vi "Cholesky decomposition LABVIEW_v1.3.vi"() -> ()   [LabVIEW 2020]
uses:
  <vilib>/Analysis/Matrix/Datatypes/RealMatrix.ctl
  <vilib>/Analysis/baseanly.llb/Real A x B.vi
  <vilib>/Analysis/7linalg.llb/Real Cholesky Factorization.vi
  <vilib>/Analysis/7linalg.llb/Real Transpose Matrix.vi
  <vilib>/Analysis/baseanly.llb/Full Cholesky Factorization.vi
  <vilib>/Analysis/baseanly.llb/Full Real Matrix Cholesky Factorization.vi
  <vilib>/Analysis/Matrix/Numeric/Subtract/Subtract - RM,RM.vi
  <vilib>/Analysis/NI_AALPro.lvlib
  <vilib>/Analysis/Matrix/NI_Matrix.lvlib
  <vilib>/Analysis/NI_AALBase.lvlib
panel:
  out "sum of error":dbl
  out "error":i32
  out "L LABVIEW-FPGA":sgl[][](array[numeric])
  out "L LABVIEW":T1
  out "A input":dbl[][](array[numeric])
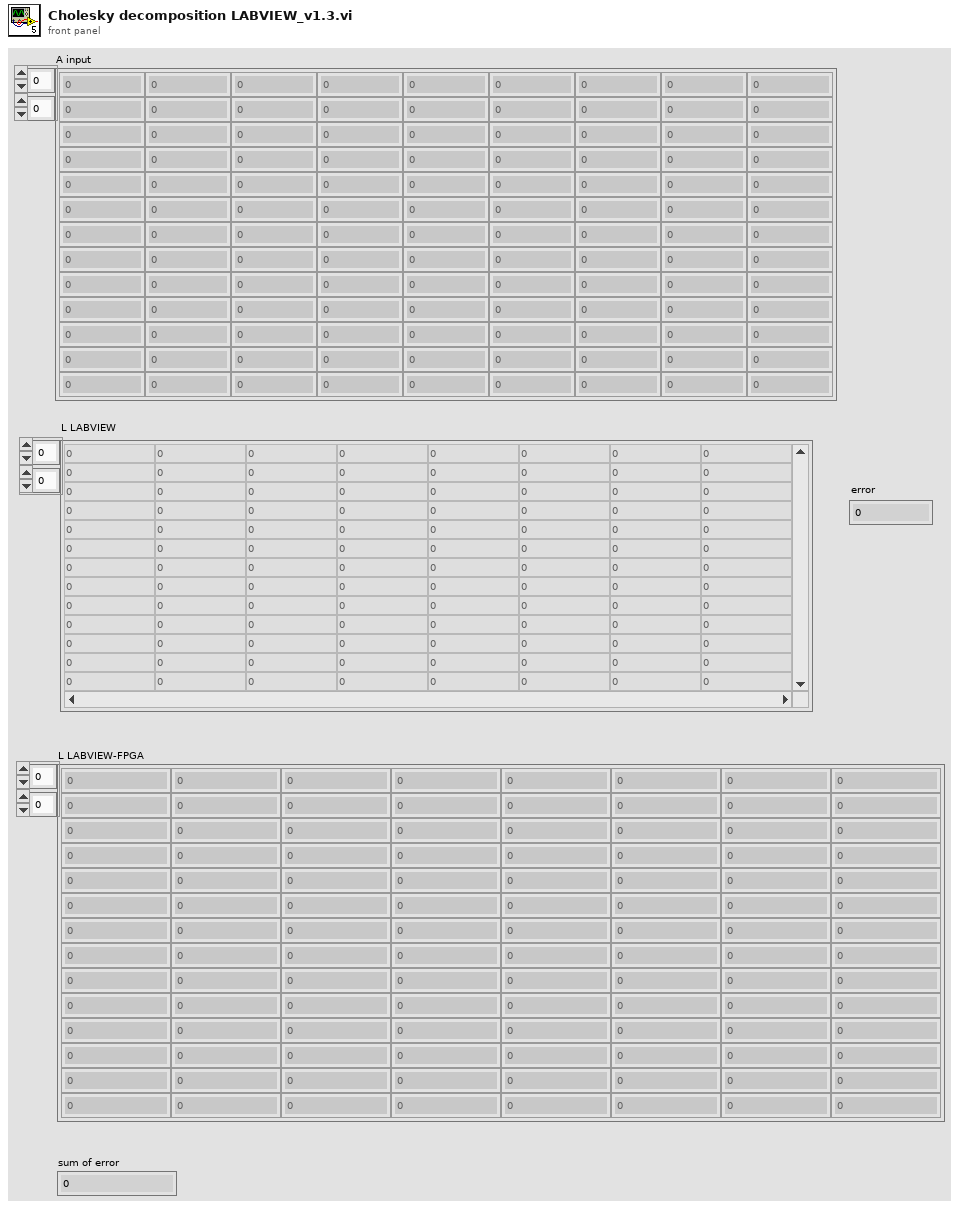
[diagram p1: front panel]
types:
  T1 = typedef "NI_Matrix.lvlib/RealMatrix.ctl" = dbl[][]
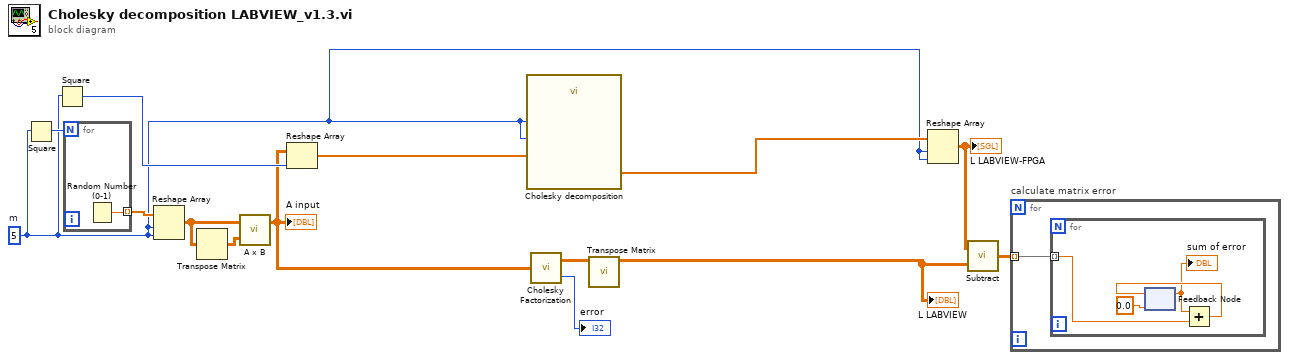
[diagram p0: block diagram]
diagram:
  w1 = 5  # m
  n1 = Square(x=w1) -> (x^2=w6:i32)
  n2 = Square(x=w1) -> (x^2=w11:i32)
  n3 = for {
    N: w6 -> [_]
    tunnel: [w15] -> w5 mode=indexing
    n4 = Random Number (0-1)() -> (number: 0 to 1=w15:dbl)
  }
  n5 = Reshape Array(w5, w1, w1) -> (w3:dbl[][])
  n6 = Transpose Matrix(1:w3) -> (0:w4:dbl[][])
  n7 = call-poly <vilib>:"A x B.vi"("B"=w4, "A"=w3) -> ("A x B"=w2:T1)  [unwired: 1 out]
  "A input" <- w2
  n8 = Reshape Array(w2, w11) -> (w14:dbl[])
  n9 = call "Cholesky decomposition.vi"("n"=w1, "m"=w1, "A"=w14) -> ("L"=w13:sgl[])
  n10 = call-poly <vilib>:"Cholesky Factorization.vi"("A"=w2) -> ("Cholesky"=w10:T1, "error"=→"error":i32)
  n11 = call-poly <vilib>:"Transpose Matrix.vi"("Input Matrix"=w10) -> ("Matrix Transpose"=w7:T1)  [unwired: 9 in, 1 out]
  "L LABVIEW" <- w7
  n12 = Reshape Array(w13, w1, w1) -> (w8:sgl[][])
  "L LABVIEW-FPGA" <- w8
  n13 = call-poly <vilib>:"Subtract.vi"("Real Matrix B"=w7, "Real Matrix A"=w8) -> ("A - B"=w9:T1)
  n14 = for "calculate matrix error" {
    tunnel: w9 -> [w16] mode=indexing
    n15 = for {
      tunnel: w16 -> [w20] mode=indexing
      n16 = feedback #1(0.0) -> (w18:dbl)
      "sum of error" <- w18
      n17 = Add(x=w18, y=w20) -> (x+y=w19:dbl)
      n18 = feedback-in #1(w19) -> ()
    }
  }
